vi "Close Device Core.vi"(8 "error in (no error)":errorcluster, 11 "IVI_DCPwr in":refnum<class "IVI_DCPwr.lvclass">) -> (0 "error out":errorcluster, 3 "IVI_DCPwr out":refnum<class "IVI_DCPwr.lvclass">)   [LabVIEW 2013, in "IVI_DCPwr.lvlib" / "IVI_DCPwr.lvclass"]
doc: "Close device driver connection."
uses:
  IVI_DCPwr.lvclass
  Base/CS++DCPwr/CS++DCPwr.lvclass
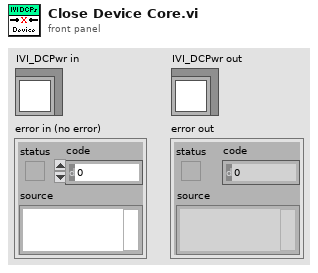
[diagram p1: front panel]
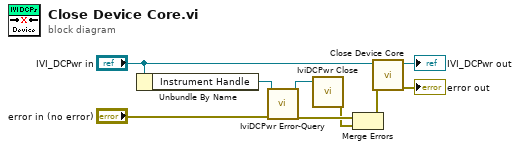
[diagram p0: block diagram]
diagram:
  n1 = Unbundle By Name("IVI_DCPwr in") -> ("Instrument Handle"=w6:refnum<k15>)
  n2 = call <vilib>:"IviDCPwr Error-Query.vi"("error in (no error)"="error in (no error)", "instrument handle"=w6) -> ("error out"=w3:errorcluster, "instrument handle out"=w5:refnum<k15>)  [unwired: 6 in, 2 out]
  n3 = call <vilib>:"IviDCPwr Close.vi"("instrument handle"=w5) -> ("error out"=w2:errorcluster)  [unwired: 10 in]
  n4 = Merge Errors(w3, w2) -> (w1:errorcluster)
  n5 = call-parent "Close Device Core.vi"("error in (no error)"=w1, "CS++DCPwr in"="IVI_DCPwr in") -> ("error out"=→"error out":errorcluster, "CS++DCPwr out"=→"IVI_DCPwr out":refnum<class "IVI_DCPwr.lvclass">)  [unwired: 8 in]
